vi "Command Pattern.vi"() -> ()   [LabVIEW 2018]
doc: "Use this template to build a producer/consumer design pattern. Use this template when you need to execute a process, such as data analysis, when a data source, such as a triggered acquisition, produces data at an uneven rate and you need to execute the process when the data becomes available."
uses:
  Message Transport_class/Message Transport.lvclass
  Message_class/Message.lvclass
  Exit_class/Exit.lvclass
  C:/GitClones/LVOOP DRAFT/Command Pattern/Action_class/Action.lvclass
  Message_class/Message.lvclass/Message.ctl
  Action_class/Action.lvclass
panel:
  in  "Do Action":bool
  in  "stop":bool
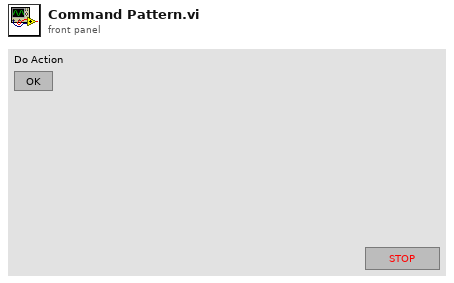
[diagram p1: front panel]
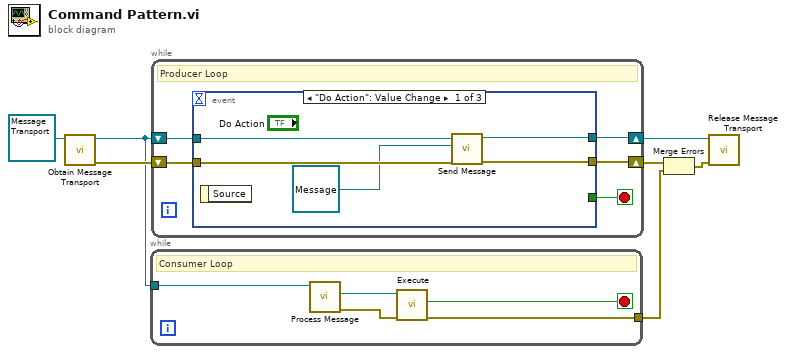
[diagram p0: block diagram]
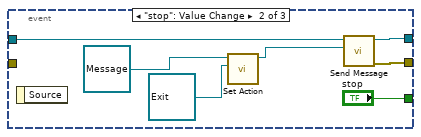
[diagram p2: hidden frame]
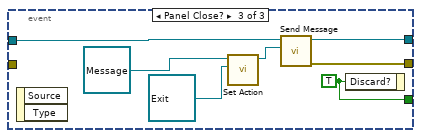
[diagram p3: hidden frame]
diagram:
  n1 = call-dynamic "Obtain Message Transport.vi"("Message Transport"=refnum<class "Message Transport.lvclass"> refnum) -> ("error out"=w5:errorcluster, "Message Transport out"=w4:refnum<class "Message Transport.lvclass">)  [unwired: 9 in]
  n2 = while {
    tunnel: w4 -> [w8]
    tunnel: [w12] -> w3
    stop <- w9 stop-if-true
    # "Consumer Loop"
    n3 = call "Process Message.vi"("Message Transport in"=w8) -> ("error out"=w10:errorcluster, "Action"=w11:refnum<class "Action.lvclass">)  [unwired: 8 in, 1 out]
    n4 = call-dynamic "Execute.vi"("error in (no error)"=w10, "Action in"=w11) -> ("error out"=w12:errorcluster, "Exit?"=w9:bool)  [unwired: 7 in, 1 out]
  }
  n5 = while {
    shift-right: [w14] -> w7
    shift-left: w5 -> [w15]
    shift-right: [w16] -> w1
    shift-left: w4 -> [w17]
    stop <- w13 stop-if-true
    # "Producer Loop"
    n6 = event shown="[0] \"Do Action\": Value Change" {
      selector: _ -> [_ _ _]
      dyn-events: _ -> [_ _ _]
      timeout: _ -> [_ _ _]
      tunnel: w17 -> [w22 w28 w36]
      tunnel: [w21 w27 w35] -> w16
      tunnel: w15 -> [w20 _ _]
      tunnel: [w19 w26 w34] -> w14
      tunnel: [_ "stop" w30] -> w13
      event "Do Action": Value Change {
        n7 = event-data() -> ()  [unwired: 1 in, 1 out]
        n8 = call "Send Message.vi"("error in (no error)"=w20, "Message.lvclass"=refnum<class "Message.lvclass"> refnum, "Message Transport in"=w22) -> ("error out"=w19:errorcluster, "Message Transport out"=w21:refnum<class "Message Transport.lvclass">)  [unwired: 7 in]
      }
      event "stop": Value Change {
        n9 = event-data() -> ()  [unwired: 1 in, 1 out]
        n10 = call "Set Action.vi"("Action"=refnum<class "Exit.lvclass"> refnum ("Message"), "Message in"=refnum<class "Message.lvclass"> refnum) -> ("Message out"=w25:refnum<class "Message.lvclass">)  [unwired: 8 in, 1 out]
        n11 = call "Send Message.vi"("Message.lvclass"=w25, "Message Transport in"=w28) -> ("error out"=w26:errorcluster, "Message Transport out"=w27:refnum<class "Message Transport.lvclass">)  [unwired: 8 in]
      }
      event Panel Close? {
        w30 = TRUE ("Discard?")
        n12 = event-data() -> ()  [unwired: 1 in, 2 out]
        n13 = call "Set Action.vi"("Action"=refnum<class "Exit.lvclass"> refnum ("Message"), "Message in"=refnum<class "Message.lvclass"> refnum) -> ("Message out"=w33:refnum<class "Message.lvclass">)  [unwired: 8 in, 1 out]
        n14 = call "Send Message.vi"("Message.lvclass"=w33, "Message Transport in"=w36) -> ("error out"=w34:errorcluster, "Message Transport out"=w35:refnum<class "Message Transport.lvclass">)  [unwired: 8 in]
        n15 = event-data("Discard?"=w30) -> ()  [unwired: 1 in, 1 out]
      }
    }
  }
  n16 = Merge Errors(w7, w3) -> (w6:errorcluster)
  n17 = call "Release Message Transport.vi"("error in (no error)"=w6, "Message Transport in"=w1) -> ()  [unwired: 10 in]
